vi "Lookup Devices by Type.vi"(8 "error in (no error)":errorcluster, 10 "Hardware Type":string, 11 "Mag Lab Measure Controller in":refnum<class "Mag Lab Measure Controller.lvclass">) -> (0 "error out":errorcluster, 2 "Matching Devices":string[](array[string]), 3 "Mag Lab Measure Controller out":refnum<class "Mag Lab Measure Controller.lvclass">)   [LabVIEW 2015, in "Mag Lab Measure Controller.lvclass"]
uses:
  Mag Lab Measure Controller.lvclass
  Mag Lab Measure Controller.lvclass/Mag Lab Measure Controller.ctl
  Mag Lab Error Handler/Mag Lab Error Handler.lvclass
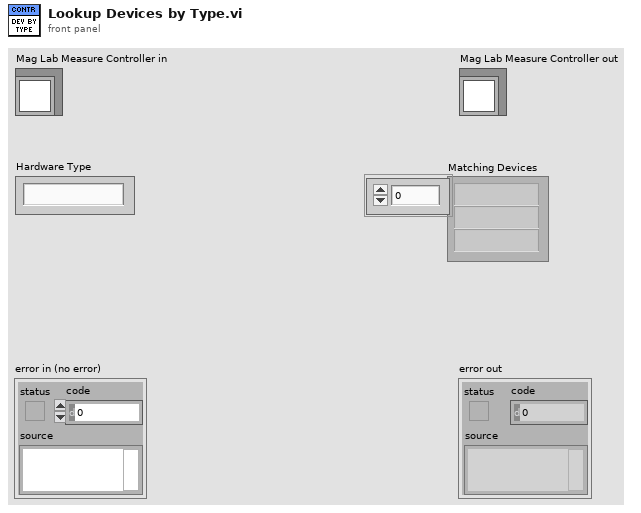
[diagram p1: front panel]
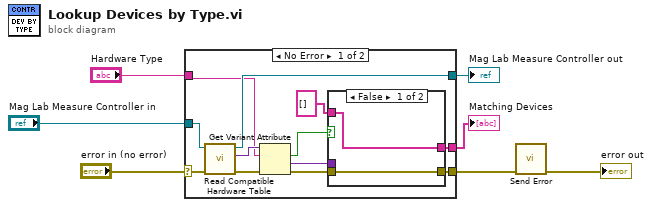
[diagram p0: block diagram]
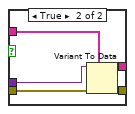
[diagram p2: hidden frame]
diagram:
  n1 = case shown="No Error" "error in (no error)" {
    selector: "error in (no error)" -> [w14 w28]
    tunnel: [w10 w28] -> w2
    tunnel: [w16 w27] -> w5
    tunnel: "Mag Lab Measure Controller in" -> [w18 w27]
    tunnel: "Hardware Type" -> [w15 _]
    tunnel: [w11 _] -> w3
    frame No Error {
      n2 = call "Read Compatible Hardware Table.vi"("error in (no error)"=w14, "Mag Lab Measure Controller in"=w18) -> ("error out"=w13:errorcluster, "Compatible Hardware Type Lookup Table (HardwareType -> DeviceNames[])"=w17:variant, "Mag Lab Measure Controller out"=w16:refnum<class "Mag Lab Measure Controller.lvclass">)  [unwired: 7 in]
      n3 = Get Variant Attribute(Variant=w17, name=w15, error in=w13) -> (found=w9:bool, value=w19:variant, error out=w12:errorcluster)  [unwired: 1 in, 1 out]
      n4 = case shown="False" w9 {
        tunnel: w19 -> [_ w26]
        tunnel: w12 -> [w20 w25]
        tunnel: [w21 w24] -> w11
        tunnel: [w20 w23] -> w10
        tunnel: string[] [] -> [w21 w22]
        frame False {
        }
        frame True {
          n5 = Variant To Data(error in=w25, type=w22, Variant=w26) -> (data=w24:string[], error out=w23:errorcluster)
        }
      }
    }
    frame Error {
    }
  }
  "Mag Lab Measure Controller out" <- w5
  "Matching Devices" <- w3
  n6 = call "Send Error.vi"("error in (no error)"=w2) -> ("error out"=→"error out":errorcluster)  [unwired: 9 in, 1 out]
